vi "test_Create Data Channel_single channel type cast.vi"(8 "error in (no error)":errorcluster, 11 "TestCase in":refnum<class "Instrument Addon Scripting API Channels Unit Tests.lvclass">) -> (0 "error out":errorcluster, 3 "TestCase out":refnum<class "Instrument Addon Scripting API Channels Unit Tests.lvclass">)   [LabVIEW 2019, in "Instrument Addon Scripting API Channels Unit Tests.lvclass"]
uses:
  Instrument Addon Scripting API Channels Unit Tests.lvclass
  APIs/Scripting API/TypeDefs/Single Channel Type Cast Settings.ctl
  Addon/Addon Shared/Types/Type Cast Type.ctl
  Addon/Addon Shared/Types/Endian.ctl
  Addon/Addon Shared/Types/Protocol Data Type.ctl
  Addon/Addon Shared/Types/Data Channel Type.ctl
  Instrument Addon Scripting API Channels Unit Tests.lvclass/Instrument Addon Scripting API Channels Unit Tests.ctl
  Addon/Addon Shared/SubVIs/Constants.vi
  <vilib>/NI/NI VeriStand Advanced SysDef API/_SubVIs/SysDef.Search.GUID.vi
  <vilib>/NI VeriStand/Custom Device API/Get Item Property (U16).vi
  APIs/Scripting API/Channels/Create Data Channel - Single Channel - Type Cast.vi
  <vilib>/NI/NI VeriStand Advanced SysDef API/_SubVIs/SysDef.Search.GUIDs.vi
  <vilib>/addons/_JKI Toolkits/VI Tester/TestCase.llb/TestCase.lvclass
  <vilib>/NI/NI VeriStand Advanced SysDef API/SysDef API/Advanced System Definition.lvlib
  Addon/Addon Shared/Instrument Addon Shared.lvlib
  <vilib>/NI VeriStand/Custom Device API/Custom Device API.lvlib
  APIs/Scripting API/Instrument Addon Scripting API.lvlib
  C:/Program Files (x86)/National Instruments/LabVIEW 2019/vi.lib/addons/_JKI Toolkits/VI Tester/TestCase.llb/TestCase.lvclass
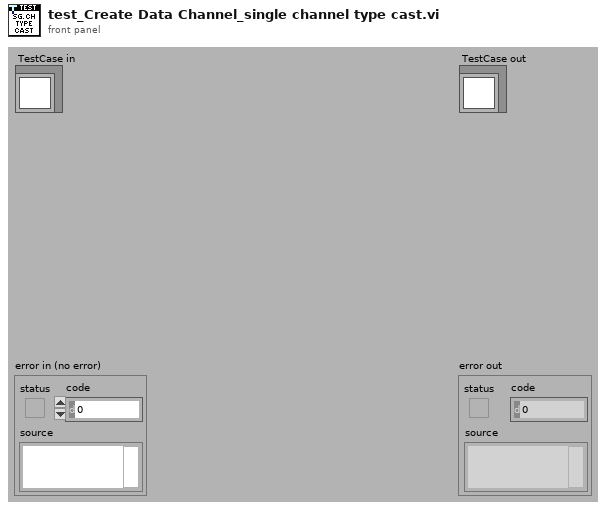
[diagram p1: front panel]
types:
  T1 = typedef "Instrument Addon Scripting API.lvlib/Single Channel Type Cast Settings.ctl" = cluster{"Default Value":dbl, "Units":string, "Type":T2, "Endian":T3}
  T2 = typedef "Instrument Addon Shared.lvlib/Type Cast Type.ctl" = enum16{"DBL", "SGL", "U64", "U32", "U16", "U8", "I64", "I32", "I16", "I8"}
  T3 = typedef "Instrument Addon Shared.lvlib/Endian.ctl" = enum16{"Native", "Little", "Big"}
  T4 = typedef "Instrument Addon Shared.lvlib/Data Channel Type.ctl" = enum16{"Format", "Comparison", "Type Cast", "Enumerated List"}
  T5 = typedef "Instrument Addon Shared.lvlib/Protocol Data Type.ctl" = enum16{"Single Channel", "Array"}
  T6 = typedef "Custom Device API.lvlib/Custom Device Item Ref.ctl" = u64
  T7 = typedef "Custom Device API.lvlib/Custom Device Channel.ctl" = cluster{"Type":T8, "Units":string, "Default Value":dbl, "Faultable":bool, "Scalable":bool}
  T8 = typedef "Custom Device API.lvlib/Custom Device Channel Type.ctl" = enum16{"Input", "Output"}
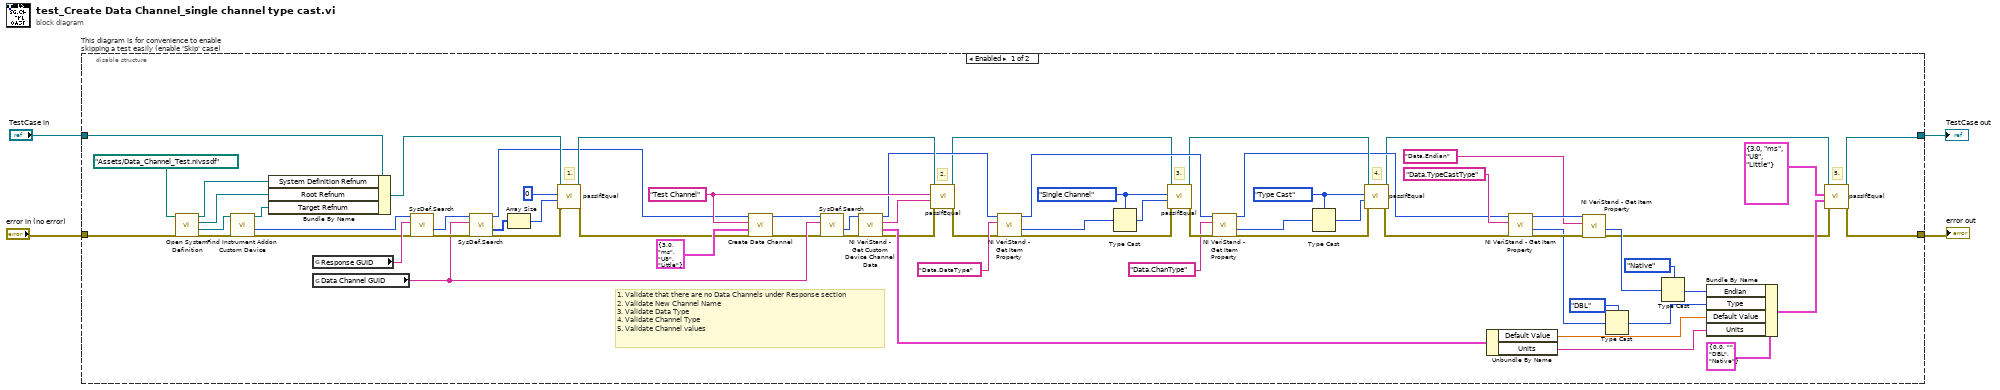
[diagram p0: block diagram]
diagram:
  n1 = disable-structure "This diagram is for convenience to enable skipping a test easily (enable 'Skip' case)" shown="Enabled" {
    disable-tunnel: "TestCase in" -> [w35 w76]
    disable-tunnel: [w72 w74] -> w1
    disable-tunnel: [w71 w75] -> w3
    disable-tunnel: "error in (no error)" -> [w67 w73]
    frame Enabled {
      w17 = Data_Channel_Type."Type Cast" ("Channel Type")
      w22 = Protocol_Data_Type."Single Channel" ("Data Type")
      w52 = "Test Channel" ("Name")
      # "2."
      # "4."
      # "3."
      # "5."
      # "1. Validate that there are no Data Channels under Response section\n2. Validate New Channel Name\n3. Validate Data Type\n4. Validate Channel Type\n5. Validate Channel values"
      # "1."
      n2 = call "Open System Definition.vi"("error in (no error)"=w67, "System Definition File"=path "Assets/Data_Channel_Test.nivssdf") -> ("error out"=w70:errorcluster, "Target Refnum"=w69:refnum<k24>, "Root Refnum"=w32:refnum<k24>, "System Definition Refnum"=w34:refnum<k24>)  [unwired: 6 in]
      n3 = call "Find Instrument Addon Custom Device.vi"("error in"=w70, "target in"=w69) -> ("error out"=w36:errorcluster, "NodeID"=w29:u64, "target out"=w31:refnum<k24>)  [unwired: 7 in]
      n4 = Bundle By Name(cluster=w35, "System Definition Refnum"=w34, "Root Refnum"=w32, "Target Refnum"=w31) -> (w33:refnum<class "Instrument Addon Scripting API Channels Unit Tests.lvclass">)
      n5 = global read "Constants.vi" "Response GUID"() -> (w66:string)
      n6 = global read "Constants.vi" "Data Channel GUID"() -> (w64:string)
      n7 = call-poly <vilib>:"SysDef.Search.vi"("error in (no error)"=w36, "GUID"=w66, "nodeID"=w29) -> ("error out"=w65:errorcluster, "Value out"=w6:u64)  [unwired: 5 in, 2 out]
      n8 = call-poly <vilib>:"SysDef.Search.vi"("error in (no error)"=w65, "GUID"=w64, "nodeID"=w6) -> ("error out"=w56:errorcluster, "Values Out"=w55:u64[], "nodeID out"=w5:u64)  [unwired: 5 in, 1 out]
      n9 = Array Size(array=w55) -> (size(s)=w54:i32)
      n10 = call-dynamic "passIfEqual.vi"("error in (no error)"=w56, "y"=w54, "x"=0 ("size(s)"), "TestCase in"=w33) -> ("error out"=w30:errorcluster, "TestCase out"=w28:refnum<class "Instrument Addon Scripting API Channels Unit Tests.lvclass">)  [unwired: 6 in]
      n11 = call-poly "Create Data Channel.vi"("error in (no error)"=w30, "settings"=T1 {"Default Value"=3.0, "Units"="ms", "Type"=enum."U8", "Endian"=enum."Little"} ("Settings"), "channel name"=w52, "response refnum in"=w5) -> ("error out"=w50:errorcluster, "response refnum out"=w51:T6)  [unwired: 5 in, 1 out]
      n12 = call-poly <vilib>:"SysDef.Search.vi"("error in (no error)"=w50, "GUID"=w64, "nodeID"=w51) -> ("error out"=w63:errorcluster, "Value out"=w38:u64)  [unwired: 5 in, 2 out]
      n13 = call <vilib>:"NI VeriStand - Get Custom Device Channel Data.vi"("error in (no error)"=w63, "Channel Ref in"=w38) -> ("error out"=w27:errorcluster, "Channel"=w62:T7, "Channel Name"=w58:string, "Channel Ref out"=w14:T6)  [unwired: 4 in, 2 out]
      n14 = call-dynamic "passIfEqual.vi"("error in (no error)"=w27, "y"=w58, "x"=w52, "TestCase in"=w28) -> ("error out"=w13:errorcluster, "TestCase out"=w12:refnum<class "Instrument Addon Scripting API Channels Unit Tests.lvclass">)  [unwired: 6 in]
      n15 = call-poly <vilib>:"NI VeriStand - Get Item Property.vi"("error in (no error)"=w13, "Property Name"="Data.DataType", "Item Ref in"=w14) -> ("error out"=w25:errorcluster, "Value"=w24:u16, "Item Ref out"=w16:T6)  [unwired: 5 in, 1 out]
      n16 = Type Cast(type=w22, x=w24) -> (*(type *) &x=w23:T5)
      n17 = call-dynamic "passIfEqual.vi"("error in (no error)"=w25, "y"=w23, "x"=w22, "TestCase in"=w12) -> ("error out"=w21:errorcluster, "TestCase out"=w11:refnum<class "Instrument Addon Scripting API Channels Unit Tests.lvclass">)  [unwired: 6 in]
      n18 = call-poly <vilib>:"NI VeriStand - Get Item Property.vi"("error in (no error)"=w21, "Property Name"="Data.ChanType", "Item Ref in"=w16) -> ("error out"=w20:errorcluster, "Value"=w19:u16, "Item Ref out"=w10:T6)  [unwired: 5 in, 1 out]
      n19 = Type Cast(type=w17, x=w19) -> (*(type *) &x=w18:T4)
      n20 = call-dynamic "passIfEqual.vi"("error in (no error)"=w20, "y"=w18, "x"=w17, "TestCase in"=w11) -> ("error out"=w9:errorcluster, "TestCase out"=w8:refnum<class "Instrument Addon Scripting API Channels Unit Tests.lvclass">)  [unwired: 6 in]
      n21 = Unbundle By Name(w62) -> ("Default Value"=w61:dbl, "Units"=w60:string)
      n22 = call-poly <vilib>:"NI VeriStand - Get Item Property.vi"("error in (no error)"=w9, "Property Name"="Data.TypeCastType", "Item Ref in"=w10) -> ("error out"=w46:errorcluster, "Value"=w40:u16, "Item Ref out"=w47:T6)  [unwired: 5 in, 1 out]
      n23 = call-poly <vilib>:"NI VeriStand - Get Item Property.vi"("error in (no error)"=w46, "Property Name"="Data.Endian", "Item Ref in"=w47) -> ("error out"=w7:errorcluster, "Value"=w43:u16)  [unwired: 5 in, 2 out]
      n24 = Type Cast(type=Type_Cast_Type."DBL" ("Type"), x=w40) -> (*(type *) &x=w39:T2)
      n25 = Type Cast(type=Endian."Native" ("Endian"), x=w43) -> (*(type *) &x=w42:T3)
      n26 = Bundle By Name(cluster=T1 {"Default Value"=0.0, "Units"="", "Type"=enum."DBL", "Endian"=enum."Native"} ("Settings"), "Endian"=w42, "Type"=w39, "Default Value"=w61, "Units"=w60) -> (w57:T1)
      n27 = call-dynamic "passIfEqual.vi"("error in (no error)"=w7, "y"=w57, "x"=T1 {"Default Value"=3.0, "Units"="ms", "Type"=enum."U8", "Endian"=enum."Little"} ("Settings"), "TestCase in"=w8) -> ("error out"=w71:errorcluster, "TestCase out"=w72:refnum<class "Instrument Addon Scripting API Channels Unit Tests.lvclass">)  [unwired: 6 in]
    }
    frame Disabled {
      # "skip test result while test is under development"
      n28 = call <vilib>:"skip.vi"("error in (no error)"=w73, "TestCase in"=w76) -> ("error out"=w75:errorcluster, "TestCase out"=w74:refnum<class "Instrument Addon Scripting API Channels Unit Tests.lvclass">)  [unwired: 8 in]
    }
  }
  "error out" <- w3
  "TestCase out" <- w1
